vi "Activity_3.vi"() -> ()   [LabVIEW 2015]
uses:
  <vilib>/measure/NI_MABase.lvlib
panel:
  in  "stop":bool
  in  "Tab Control":T1(tab)=enum."Suma de Señales"
  in  "Numeric":dbl=1.0
  in  "Numeric 2":dbl=2.0
  out "Numeric 3":dbl=3.0
  in  "Array":dbl[](array[numeric])=[1.0, 2.0, 3.0, 4.0]
  in  "Numeric 4":dbl=5.0
  out "x+y":dbl[](array[numeric])
  in  "Array 2":dbl[](array[numeric])=[1.0, 2.0, 3.0, 4.0]
  in  "Array 3":dbl[](array[numeric])=[5.0, 6.0, 7.0, 8.0]
  out "x+y 2":dbl[](array[numeric])=[6.0, 8.0, 10.0, 12.0]
  out "offset":waveform(dbl)(graph)={"t0"=timestamp(104671.0 s since 1904-01-01), "dt"=0.001, "Y"=array[1000 elements]}
  out "signal out":waveform(dbl)(graph)={"t0"=timestamp(104671.0 s since 1904-01-01), "dt"=0.001, "Y"=array[1000 elements]}
  out "x":waveform(dbl)(graph)={"t0"=timestamp(104671.0 s since 1904-01-01), "dt"=0.001, "Y"=array[1000 elements]}
  # "Suma de Diferentes Tipos de Datos"
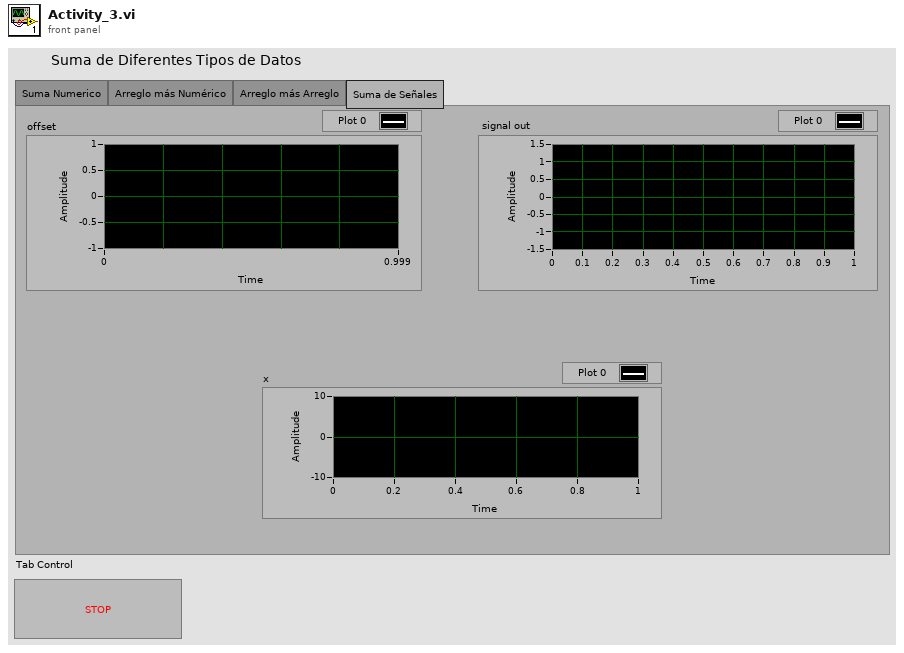
[diagram p1: front panel]
types:
  T1 = enum32{"Suma Numerico", "Arreglo más Numérico", "Arreglo más Arreglo", "Suma de Señales"}
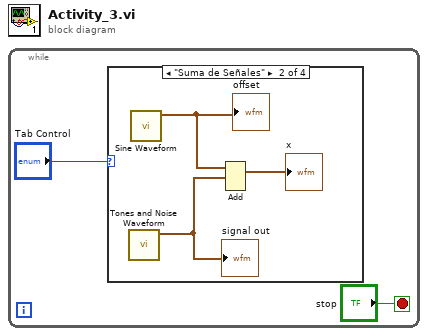
[diagram p0: block diagram]
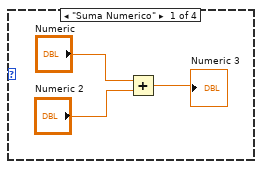
[diagram p2: hidden frame]
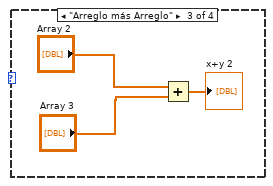
[diagram p3: hidden frame]
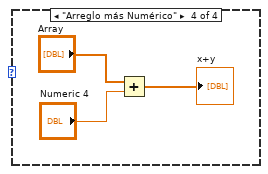
[diagram p4: hidden frame]
diagram:
  n1 = while {
    stop <- "stop" stop-if-true
    n2 = case shown="\"Suma de Señales\"" "Tab Control" {
      frame "Suma Numerico" {
        n3 = Add(x="Numeric", y="Numeric 2") -> (x+y=→"Numeric 3":dbl)
      }
      frame "Suma de Señales" {
        n4 = call <vilib>:"Tones and Noise Waveform.vi"() -> ("signal out"=w6:waveform(dbl))  [unwired: 10 in, 1 out]
        "signal out" <- w6
        n5 = call <vilib>:"Sine Waveform.vi"() -> ("signal out"=w8:waveform(dbl))  [unwired: 10 in, 1 out]
        "offset" <- w8
        n6 = Add(1:w6, 2:w8) -> (0:→"x":waveform(dbl))  [unwired: 1 in, 1 out]
      }
      frame "Arreglo más Arreglo" {
        n7 = Add(x="Array 2", y="Array 3") -> (x+y=→"x+y 2":dbl[])
      }
      frame "Arreglo más Numérico" {
        n8 = Add(x="Array", y="Numeric 4") -> (x+y=→"x+y":dbl[])
      }
    }
  }
